vi "ApplyPropertyTemplateToMethod.vi"(0 "ClassWriterNative in":refnum<class "ClassWriterNative.lvclass">, 1 "VIRef":refnum<vi>, 2 "ClassRef":refnum<vi>, 3 "PropertyName":string, 4 "MethodTemplateName":string, 5 "error in (no error)":errorcluster) -> (14 "ClassWriterNative out":refnum<class "ClassWriterNative.lvclass">, 19 "error out":errorcluster)   [LabVIEW 2012, in "ClassWriterNative.lvclass"]
uses:
  <resource>/Framework/Providers/Open_GDS/ClassProviders/Provider_LvNativeClass/ClassWriterNative_class/ClassWriterNative.lvclass
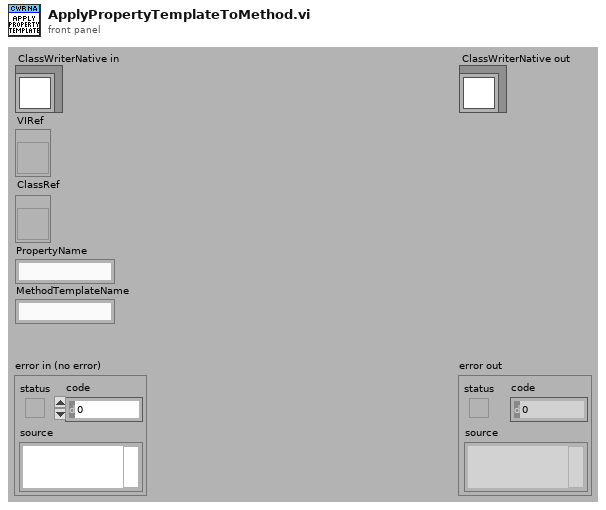
[diagram p1: front panel]
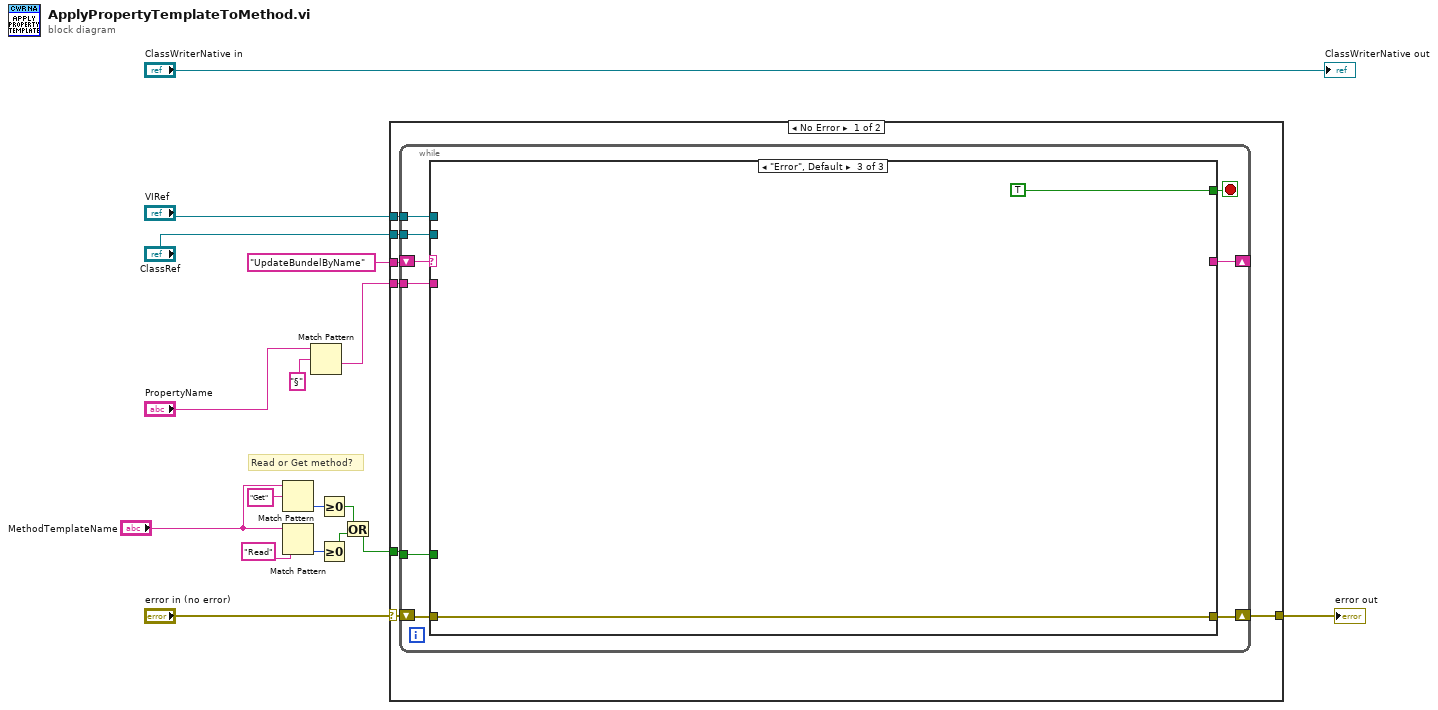
[diagram p0: block diagram]
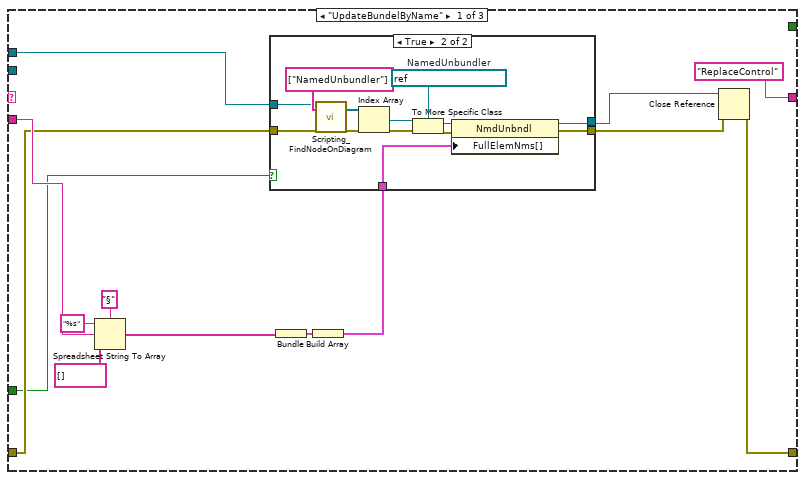
[diagram p2: hidden frame]
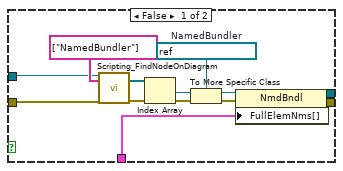
[diagram p3: hidden frame]
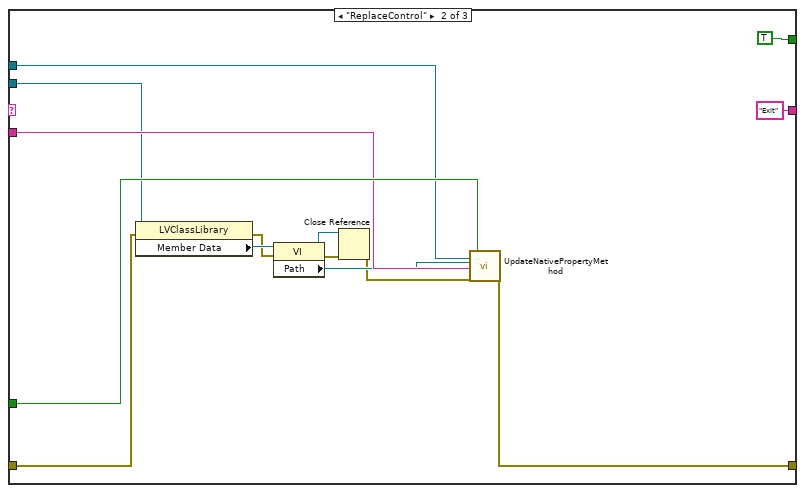
[diagram p4: hidden frame]
diagram:
  # "Read or Get method?"
  n1 = Match Pattern(string="MethodTemplateName", regular expression="Get") -> (offset past match=w5:i32)  [unwired: 1 in, 3 out]
  n2 = Match Pattern(string="MethodTemplateName", regular expression="Read") -> (offset past match=w16:i32)  [unwired: 1 in, 3 out]
  n3 = Match Pattern(string="PropertyName", regular expression="§" ("search string")) -> (after substring=w8:string)  [unwired: 1 in, 3 out]
  n4 = Greater Or Equal To 0?(x=w5) -> (x >= 0?=w3:bool)
  n5 = Greater Or Equal To 0?(x=w16) -> (x >= 0?=w4:bool)
  n6 = Or(x=w3, y=w4) -> (x .or. y?=w2:bool)
  n7 = case shown="No Error" "error in (no error)" {
    selector: "error in (no error)" -> [w18 w88]
    tunnel: "UpdateBundelByName" -> [w24 _]
    tunnel: "VIRef" -> [w23 _]
    tunnel: "ClassRef" -> [w22 _]
    tunnel: w2 -> [w21 _]
    tunnel: w8 -> [w20 _]
    tunnel: [w19 w88] -> w13
    frame No Error {
      n8 = while {
        tunnel: w23 -> [w33]
        tunnel: w20 -> [w32]
        shift-right: [w30] -> w19
        shift-left: w18 -> [w31]
        shift-right: [w28] -> _
        shift-left: w24 -> [w29]
        tunnel: w22 -> [w26]
        tunnel: w21 -> [w25]
        stop <- w27 stop-if-true
        n9 = case shown="\"Error\", Default" w29 {
          tunnel: w33 -> [w35 w81 _]
          tunnel: w32 -> [w45 w80 _]
          tunnel: w31 -> [w36 w72 w86]
          tunnel: [w47 w83 w86] -> w30
          tunnel: ["ReplaceControl" "Exit" _] -> w28
          tunnel: [_ TRUE TRUE] -> w27
          tunnel: w26 -> [_ w75 _]
          tunnel: w25 -> [w34 w82 _]
          frame "UpdateBundelByName" {
            n10 = Spreadsheet String To Array(delimiter (Tab)="§" ("search string"), format string="%s", spreadsheet string=w45, array type (2D Dbl)=string[] [] ("appended array")) -> (array=w37:string[])
            n11 = Bundle("appended array"=w37) -> (w41:cluster{"appended array":string[]})  [unwired: 1 in]
            n12 = Build Array(w41) -> (w40:cluster{"appended array":string[]}[])
            n13 = case shown="True" w34 {
              tunnel: w36 -> [w53 w69]
              tunnel: w35 -> [w52 w66]
              tunnel: w40 -> [w48 w63]
              tunnel: [w50 w61] -> w39
              tunnel: [w49 w60] -> w38
              frame False {
                w56 = refnum<vi> refnum  # NamedBundler
                n14 = call <resource>:"Scripting_FindNodeOnDiagram.vi"("ViRef(Ignored If Not Wired)"=w52, "NodeTypesToSearchFor"=string[] ["NamedBundler"], "error in (no error)"=w53) -> ("Nodes"=w54:refnum<vi>[], "error out"=w58:errorcluster)  [unwired: 15 in]
                n15 = Index Array(array=w54) -> (element=w57:refnum<vi>)  [unwired: 1 in]
                n16 = To More Specific Class(target class=w56, reference=w57, error in=w58) -> (specific class reference=w59:refnum<vi>, error out=w51:errorcluster)
                n17 = property class="NmdBndl"(reference=w59, error in=w51, "FullElemNms[]"=w48) -> (reference out=w49:refnum<vi>, error out=w50:errorcluster)
              }
              frame True {
                w62 = refnum<vi> refnum  # NamedUnbundler
                n18 = call <resource>:"Scripting_FindNodeOnDiagram.vi"("ViRef(Ignored If Not Wired)"=w66, "NodeTypesToSearchFor"=string[] ["NamedUnbundler"], "error in (no error)"=w69) -> ("Nodes"=w70:refnum<vi>[], "error out"=w68:errorcluster)  [unwired: 15 in]
                n19 = Index Array(array=w70) -> (element=w67:refnum<vi>)  [unwired: 1 in]
                n20 = To More Specific Class(target class=w62, reference=w67, error in=w68) -> (specific class reference=w65:refnum<vi>, error out=w64:errorcluster)
                n21 = property class="NmdUnbndl"(reference=w65, error in=w64, "FullElemNms[]"=w63) -> (reference out=w60:refnum<vi>, error out=w61:errorcluster)
              }
            }
            n22 = Close Reference(reference=w38, error in (no error)=w39) -> (error out=w47:errorcluster)
          }
          frame "ReplaceControl" {
            n23 = property class="LVClassLibrary"(reference=w75, error in=w72) -> (error out=w78:errorcluster, "Member Data"=w79:refnum<vi>)  [unwired: 1 out]
            n24 = property class="VI"(reference=w79, error in=w78) -> (reference out=w76:refnum<vi>, error out=w77:errorcluster, "Path"=w74:path)
            n25 = Close Reference(reference=w76, error in (no error)=w77) -> (error out=w73:errorcluster)
            n26 = call <resource>:"UpdateNativePropertyMethod.vi"("VI"=w81, "TypeDefControl"=w74, "Property"=w80, "error IO"=w73, "GetMethod"=w82) -> ("error out"=w83:errorcluster)  [unwired: 14 in]
          }
          frame "Error", Default {
          }
        }
      }
    }
    frame Error {
    }
  }
  "error out" <- w13
  "ClassWriterNative out" <- "ClassWriterNative in"
